vi "Tablet xbox Main.vi"() -> ()   [LabVIEW 2009]
uses:
  UDP Lib/UDP Network Location.ctl
  <vilib>/Utility/inputDevices.llb/closeJoystick.vi
  <vilib>/Utility/inputDevices.llb/joystickAcquire.vi
panel:
  out "Speed":dbl(slide) scale=-128.0..128.0
  out "Radius":dbl(slide) scale=-128.0..128.0
  out "axis info":T1
  out "direction info":T2
  out "A":bool caption="Boolean"
  out "B":bool
  out "Y":bool
  out "X":bool
  out "RB":bool
  out "LB":bool
  out "LThumb":i32(slide) scale=-32768.0..32768.0
  out "Cluster":T3
  out "Left Thumb button":bool
  out "Right trigger":bool
  out "Left Trigger":bool
  out "Stop/Back":bool
  out "Start":bool
  out "R Thumb":i32(slide) scale=-32768.0..32768.0
  out "Right Thumb button":bool
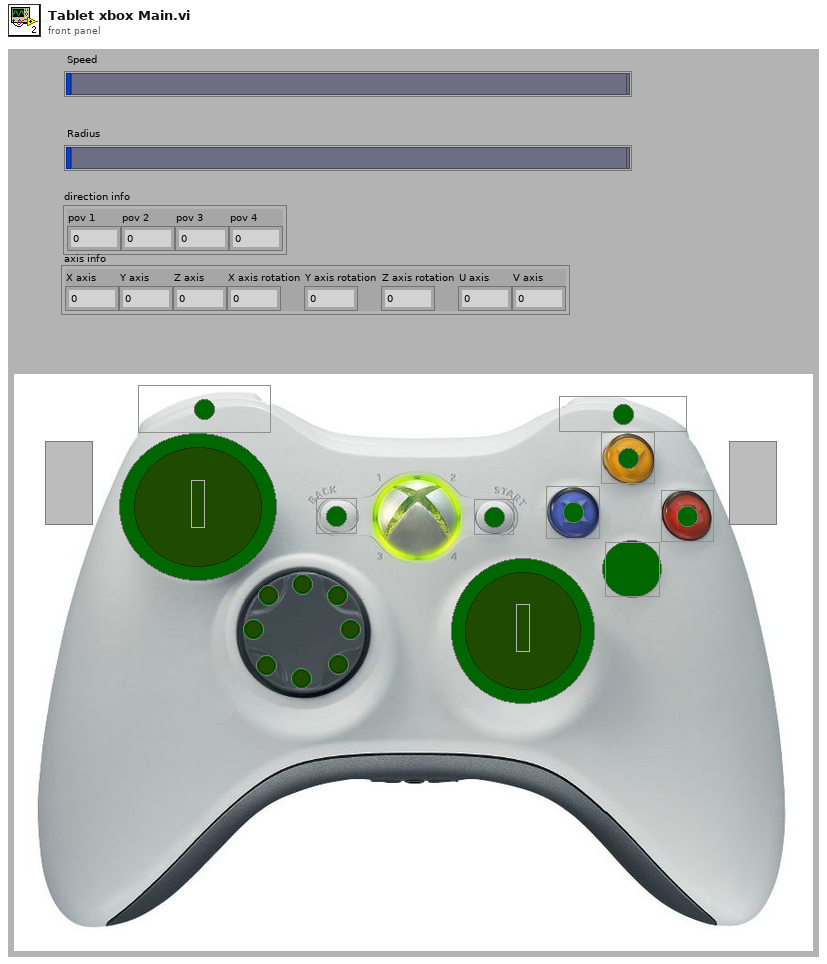
[diagram p1: front panel]
types:
  T1 = cluster{"X axis":i32, "Y axis":i32, "Z axis":i32, "X axis rotation":i32, "Y axis rotation":i32, "Z axis rotation":i32, "U axis":i32, "V axis":i32}
  T2 = cluster{"pov 1":i32, "pov 2":i32, "pov 3":i32, "pov 4":i32}
  T3 = cluster{"Boolean 4":bool, "Boolean 6":bool, "Boolean 3":bool, "Boolean 7":bool, "Boolean 2":bool, "Boolean 9":bool, "Boolean 5":bool, "Boolean 8":bool}
  T4 = typedef "UDP Base.ctl" = cluster{"UDP Session":refnum<k16>, "UDP Socket Params":T5}
  T5 = typedef "UDP Socket Params.ctl" = cluster{"Local Port":u16, "Read Timeout":i32, "Write Timeout":i32}
  T6 = typedef "UDP Network Location.ctl" = cluster{"IP Address":string, "Port":u16}
  T7 = cluster{"button 1":bool, "button 2":bool, "button 3":bool, "button 4":bool, "button 5":bool, "button 6":bool, "button 7":bool, "button 8":bool, "button 9":bool, "button 10":bool, "button 11":bool, "button 12":bool, "button 13":bool, "button 14":bool, "button 15":bool, "button 16":bool, "button 17":bool, "button 18":bool, "button 19":bool, "button 20":bool, "button 21":bool, "button 22":bool, "button 23":bool, "button 24":bool, "button 25":bool, "button 26":bool, "button 27":bool, "button 28":bool, "button 29":bool, "button 30":bool, "button 31":bool, "button 32":bool}
  T8 = cluster{"Array[0]":bool, "Array[1]":bool, "Array[2]":bool, "Array[3]":bool, "Array[4]":bool, "Array[5]":bool, "Array[6]":bool, "Array[7]":bool}
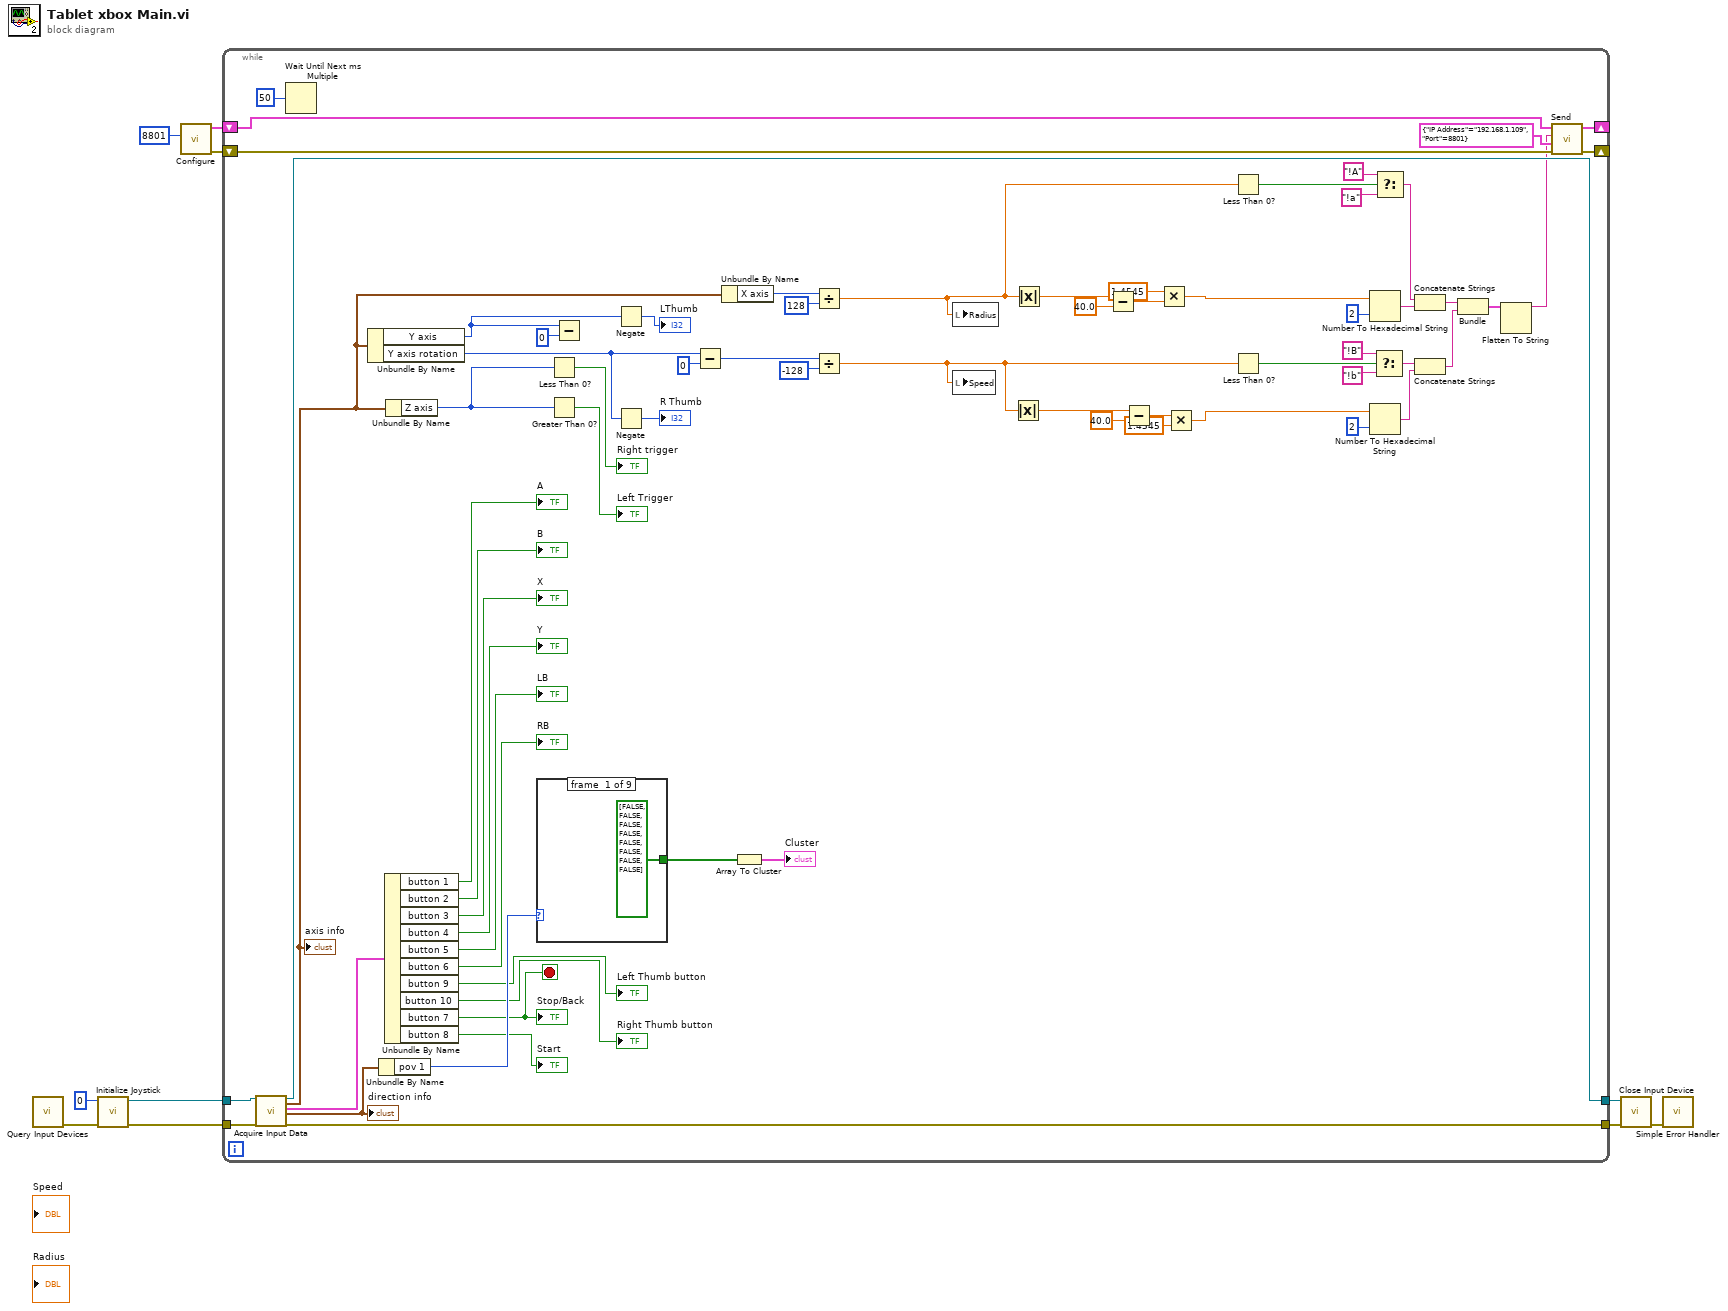
[diagram p0: block diagram]
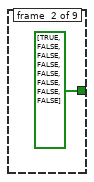
[diagram p2: hidden frame]
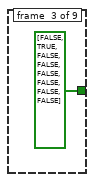
[diagram p3: hidden frame]
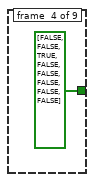
[diagram p4: hidden frame]
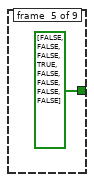
[diagram p5: hidden frame]
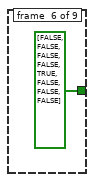
[diagram p6: hidden frame]
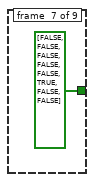
[diagram p7: hidden frame]
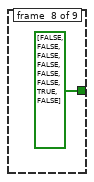
[diagram p8: hidden frame]
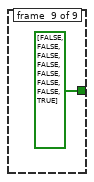
[diagram p9: hidden frame]
diagram:
  n1 = call <vilib>:"Query Input Devices.vi"() -> ("error out"=w5:errorcluster)  [unwired: 1 in, 10 out]
  n2 = call <vilib>:"Initialize Joystick.vi"("error in (no error)"=w5, "device index"=0) -> ("error out"=w8:errorcluster, "device ID"=w9:refnum<k1>)  [unwired: 8 out]
  n3 = call "Configure.vi"("Local Port"=u16 8801) -> ("error out"=w2:errorcluster, "UDP Base out"=w1:T4)  [unwired: 9 in]
  n4 = while {
    tunnel: w9 -> [w77]
    tunnel: w8 -> [w76]
    tunnel: [w75] -> w7
    tunnel: [w59] -> w6
    shift-right: [w41] -> _
    shift-left: w1 -> [w42]
    shift-right: [w40] -> _
    shift-left: w2 -> [w44]
    stop <- w57 stop-if-true
    n5 = call-poly <vilib>:"Acquire Input Data.vi"("device ID"=w77, "error in (no error)"=w76) -> ("device ID"=w75:refnum<k1>, "axis info"=w46:T1, "button info"=w74:T7, "direction info"=w68:T2, "error out"=w59:errorcluster)  [unwired: 13 out]
    "axis info" <- w46
    "direction info" <- w68
    n6 = Wait Until Next ms Multiple(millisecond multiple=u32 50) -> ()  [unwired: 1 out]
    n7 = Unbundle By Name(w46) -> ("Y axis"=w48:i32, "Y axis rotation"=w19:i32)
    n8 = Unbundle By Name(w68) -> ("pov 1"=w67:i32)
    n9 = Unbundle By Name(w74) -> ("button 1"=→"A":bool, "button 2"=→"B":bool, "button 3"=→"X":bool, "button 4"=→"Y":bool, "button 5"=→"LB":bool, "button 6"=→"RB":bool, "button 9"=→"Left Thumb button":bool, "button 10"=→"Right Thumb button":bool, "button 7"=w57:bool, "button 8"=→"Start":bool)
    "Stop/Back" <- w57
    n10 = Unbundle By Name(w46) -> ("Z axis"=w62:i32)
    n11 = case shown="-1, Default" w67 {
      tunnel: [bool[] [FALSE, FALSE, FALSE, FALSE, FALSE, FALSE, FALSE, FALSE] ("Array") bool[] [TRUE, FALSE, FALSE, FALSE, FALSE, FALSE, FALSE, FALSE] ("Array") bool[] [FALSE, TRUE, FALSE, FALSE, FALSE, FALSE, FALSE, FALSE] ("Array") bool[] [FALSE, FALSE, TRUE, FALSE, FALSE, FALSE, FALSE, FALSE] ("Array") bool[] [FALSE, FALSE, FALSE, TRUE, FALSE, FALSE, FALSE, FALSE] ("Array") bool[] [FALSE, FALSE, FALSE, FALSE, TRUE, FALSE, FALSE, FALSE] ("Array") bool[] [FALSE, FALSE, FALSE, FALSE, FALSE, TRUE, FALSE, FALSE] ("Array") bool[] [FALSE, FALSE, FALSE, FALSE, FALSE, FALSE, TRUE, FALSE] ("Array") bool[] [FALSE, FALSE, FALSE, FALSE, FALSE, FALSE, FALSE, TRUE] ("Array")] -> w66
      frame #0 {
      }
      frame #1 {
      }
      frame #2 {
      }
      frame #3 {
      }
      frame #4 {
      }
      frame #5 {
      }
      frame #6 {
      }
      frame #7 {
      }
      frame #8 {
      }
    }
    n12 = Less Than 0?(x=w62) -> (x < 0?=→"Right trigger":bool)
    n13 = Greater Than 0?(x=w62) -> (x > 0?=→"Left Trigger":bool)
    n14 = Subtract(x=w48, y=0) -> ()  [unwired: 1 out]
    n15 = Negate(x=w48) -> (-x=→"LThumb":i32)
    n16 = Negate(x=w19) -> (-x=→"R Thumb":i32)
    n17 = Subtract(x=w19, y=0) -> (x-y=w49:i32)
    n18 = Unbundle By Name(w46) -> ("X axis"=w45:i32)
    n19 = Array To Cluster(array=w66) -> (cluster=→"Cluster":T8)
    n20 = Divide(x=w45, y=128) -> (x/y=w25:dbl)
    n21 = Divide(x=w49, y=-128) -> (x/y=w24:dbl)
    n22 = local write "Radius"(w25) -> ()
    n23 = local write "Speed"(w24) -> ()
    n24 = Absolute Value(x=w24) -> (abs(x)=w39:dbl)
    n25 = Absolute Value(x=w25) -> (abs(x)=w38:dbl)
    n26 = Subtract(x=w38, y=40.0) -> (x-y=w18:dbl)
    n27 = Subtract(x=w39, y=40.0) -> (x-y=w16:dbl)
    n28 = Multiply(x=1.4545, y=w18) -> (x*y=w14:dbl)
    n29 = Multiply(x=w16, y=1.4545) -> (x*y=w13:dbl)
    n30 = Less Than 0?(x=w25) -> (x < 0?=w31:bool)
    n31 = Less Than 0?(x=w24) -> (x < 0?=w36:bool)
    n32 = Number To Hexadecimal String(1:i16 2 ("width (-)"), 2:w14) -> (0:w28:string)
    n33 = Number To Hexadecimal String(1:i16 2 ("width (-)"), 2:w13) -> (0:w23:string)
    n34 = Select(t="!B", s=w36, f="!b") -> (s? t:f=w30:string)
    n35 = Select(t="!A", s=w31, f="!a") -> (s? t:f=w29:string)
    n36 = Concatenate Strings(w29, w28) -> (w27:string)
    n37 = Concatenate Strings(w30, w23) -> (w26:string)
    n38 = Bundle(w27, w26) -> (w21:cluster{string, string})  [unwired: 1 in]
    n39 = Flatten To String(anything=w21) -> (data string=w20:string)  [unwired: 3 in, 2 out]
    n40 = call "Send.vi"("error in (no error)"=w44, "Destination Location"=T6 {"IP Address"="192.168.1.109", "Port"=8801}, "Send Data"=w20, "UDP Base in"=w42) -> ("error out"=w40:errorcluster, "UDP Base out"=w41:T4)  [unwired: 5 in, 1 out]
  }
  n41 = call-poly <vilib>:"Close Input Device.vi"("error in (no error)"=w6, "device ID"=w7) -> ("error out"=w4:errorcluster)  [unwired: 8 out]
  n42 = call <vilib>:"Simple Error Handler.vi"("error in (no error)"=w4) -> ()  [unwired: 1 in, 8 out]
